vi "TestThreshold.vi"() -> ()   [LabVIEW 2017]
panel:
  out "Image 2":T1(plugin-control)
  out "Image":T1(plugin-control)
  in  "Threshold Value":sgl=1.0 format="%.2f"
  out "error out":errorcluster
  in  "error in (no error)":errorcluster
  in  "File Path":path
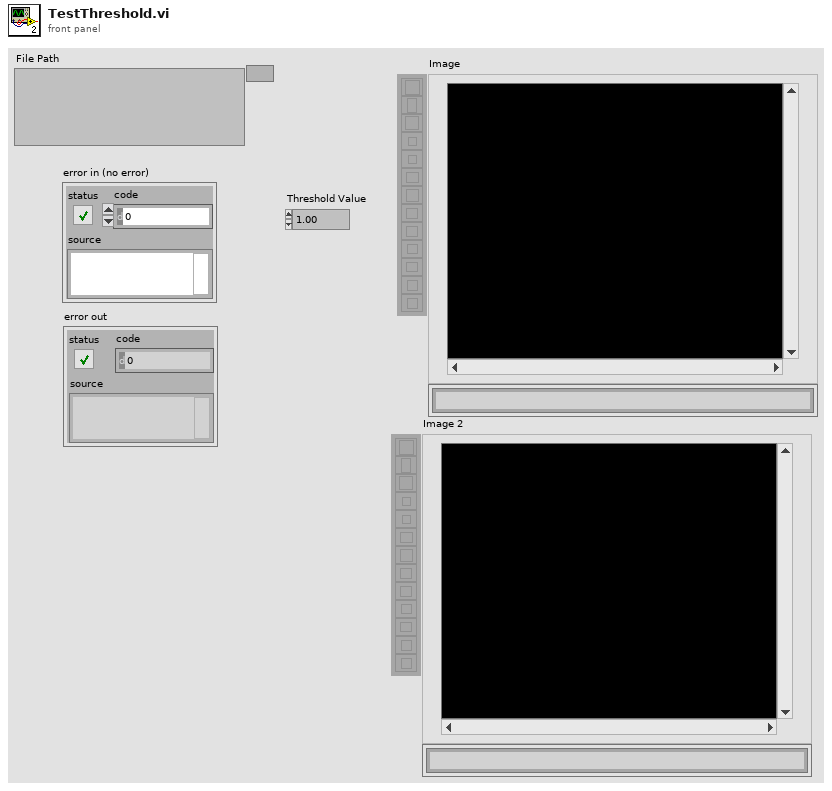
[diagram p1: front panel]
types:
  T1 = typedef "IMAQ Image.ctl" = refnum<image>
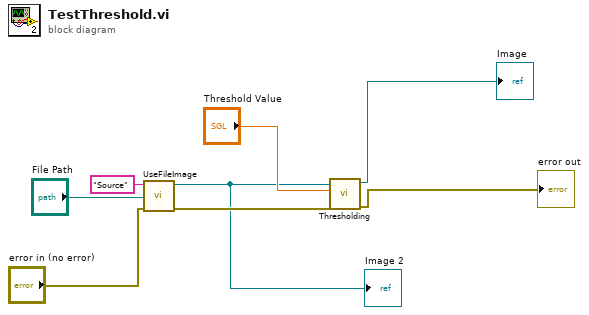
[diagram p0: block diagram]
diagram:
  n1 = call "UseFileImage.vi"("error in (no error)"="error in (no error)", "File Path"="File Path", "Image Name"="Source") -> ("error out"=w5:errorcluster, "Original Image"=w1:T1)  [unwired: 7 in]
  "Image 2" <- w1
  n2 = call "Thresholding.vi"("error in (no error)"=w5, "Threshold Value"="Threshold Value", "Image Src"=w1) -> ("error out"=→"error out":errorcluster, "Image"=→"Image":T1)  [unwired: 7 in]
